vi "Check Limits.vi"(9 "Has Lower":T2, 10 "Limits Data":T3) -> (2 "Limit State":T1)   [LabVIEW 2013, in "Limits X.xctl"]
uses:
  Limits X.xctl
  Limits Data.ctl
  lib/Apps/Yes No Button.ctl
  lib/Limits/Limite State.ctl
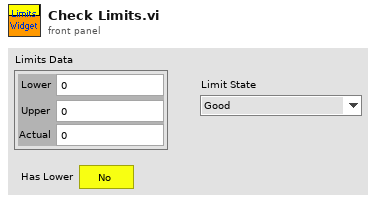
[diagram p1: front panel]
types:
  T1 = typedef "Limite State.ctl" = enum16{"Good", "Lower Bound Fault", "Upper Bound Fault"}
  T2 = typedef "Yes No Button.ctl" = bool
  T3 = typedef "Limits X.xctl/Limits Data.ctl" = cluster{"Lower":dbl, "Upper":dbl, "Actual":dbl}
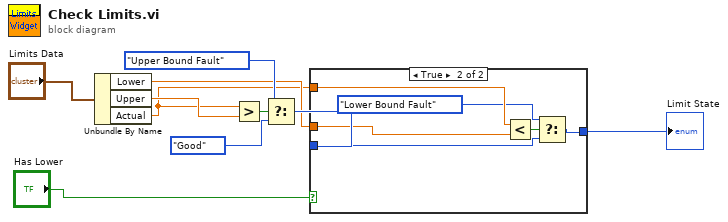
[diagram p0: block diagram]
diagram:
  n1 = Unbundle By Name("Limits Data") -> ("Lower"=w4:dbl, "Upper"=w3:dbl, "Actual"=w1:dbl)
  n2 = Greater?(x=w1, y=w3) -> (0:w8:bool)
  n3 = Select(t=Limite_State."Upper Bound Fault", s=w8, f=Limite_State."Good" ("Limit State")) -> (s? t:f=w5:T1)
  n4 = case shown="True" "Has Lower" {
    tunnel: w5 -> [w11 w16]
    tunnel: w4 -> [_ w15]
    tunnel: w1 -> [_ w14]
    tunnel: [w11 w12] -> w2
    frame False {
    }
    frame True {
      n5 = Less?(x=w14, y=w15) -> (x < y?=w17:bool)
      n6 = Select(t=Limite_State."Lower Bound Fault", s=w17, f=w16) -> (s? t:f=w12:T1)
    }
  }
  "Limit State" <- w2
